vi "WriteTextFile.vi"(8 "error in":errorcluster caption="错误输入", 10 "FilePath":string, 11 "TextIn":string) -> (0 "error out":errorcluster caption="错误输出", 3 "PathOut":path)   [LabVIEW 2013]
panel:
  out "MD5 message-digest":string caption="MD5信息摘要"
  out "长度":i32
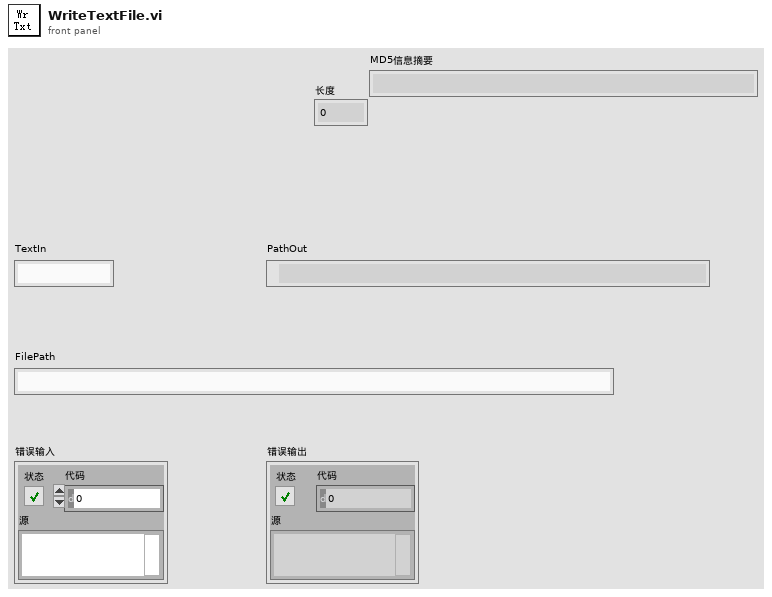
[diagram p1: front panel]
types:
  T1 = enum16{"open", "replace", "create", "open or create", "replace or create", "replace or create with confirmation"}
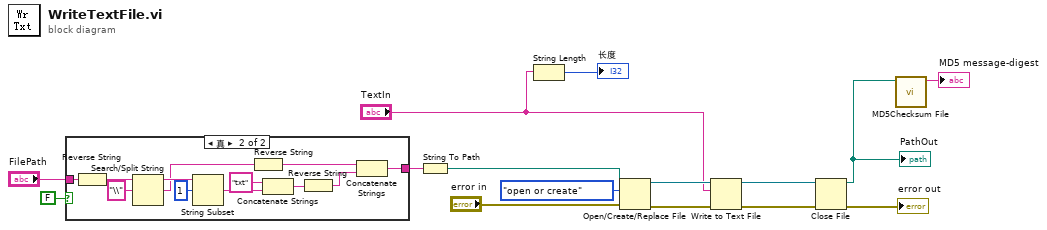
[diagram p0: block diagram]
diagram:
  n1 = case shown="真" FALSE {
    tunnel: "FilePath" -> [w16 w18]
    tunnel: [w16 w17] -> w2
    frame False {
    }
    frame True {
      n2 = Reverse String(1:w18) -> (0:w28:string)
      n3 = Search/Split String(string=w28, search string/char (-)="\\") -> (substring before match=w26:string, match + rest of string=w21:string)  [unwired: 1 in, 1 out]
      n4 = String Subset(string=w26, offset (0)=1) -> (substring=w24:string)  [unwired: 1 in]
      n5 = Reverse String(1:w21) -> (0:w20:string)
      n6 = Concatenate Strings("txt", w24) -> (w22:string)
      n7 = Reverse String(1:w22) -> (0:w19:string)
      n8 = Concatenate Strings(w20, w19) -> (w17:string)
    }
  }
  n9 = String To Path(string=w2) -> (path=w14:path)
  n10 = String Length(string="TextIn") -> (length=→"长度":i32)
  n11 = Open/Create/Replace File(file path (use dialog)=w14, error in="error in", operation (0:open)=T1."open or create" ("操作(0:open)")) -> (refnum out=w13:refnum<file>, error out=w12:errorcluster)  [unwired: 3 in, 1 out]
  n12 = Write to Text File(file (use dialog)=w13, text="TextIn", error in=w12) -> (refnum out=w11:refnum<file>, error out=w10:errorcluster)  [unwired: 1 in, 1 out]
  n13 = Close File(refnum=w11, error in=w10) -> (path=w5:path, error out=→"error out":errorcluster)
  "PathOut" <- w5
  n14 = call <vilib>:"MD5Checksum File.vi"("Path"=w5) -> ("MD5 message-digest"=→"MD5 message-digest":string)  [unwired: 9 in, 1 out]
